vi "produceTimingTicks.vi"(8 "error in (no error)":errorcluster, 10 "Channel":refnum<class "Channel.lvclass">, 11 "RampEvent in":refnum<class "RampEvent.lvclass">) -> (0 "error out":errorcluster, 2 "timingTickList":refnum<class "ScriptEventList.lvclass">, 3 "RampEvent out":refnum<class "RampEvent.lvclass">)   [LabVIEW 2011, in "Tools.lvlib" / "Scripting.lvlib" / "RampEvent.lvclass"]
uses:
  RampEvent.lvclass
  DatabaseHelpers/Database Objects/Channel/Channel.lvclass
  ScriptEventList/ScriptEventList.lvclass
  ScriptEvent.lvclass
panel:
  out "Array":dbl[](array[numeric]) format="%_10g"
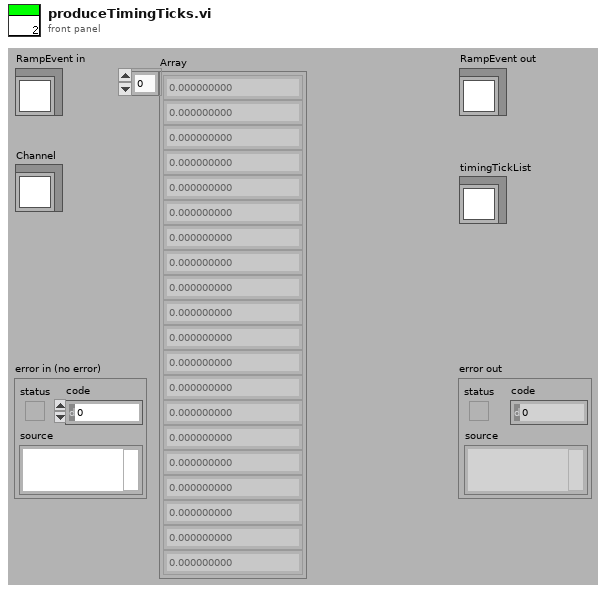
[diagram p1: front panel]
types:
  T1 = enum16{"changeValue", "pulse", "clock", "rampUp", "rampDown", "singleTone", "singleToneRamp", "playFile", "rf", "rfRamp"}
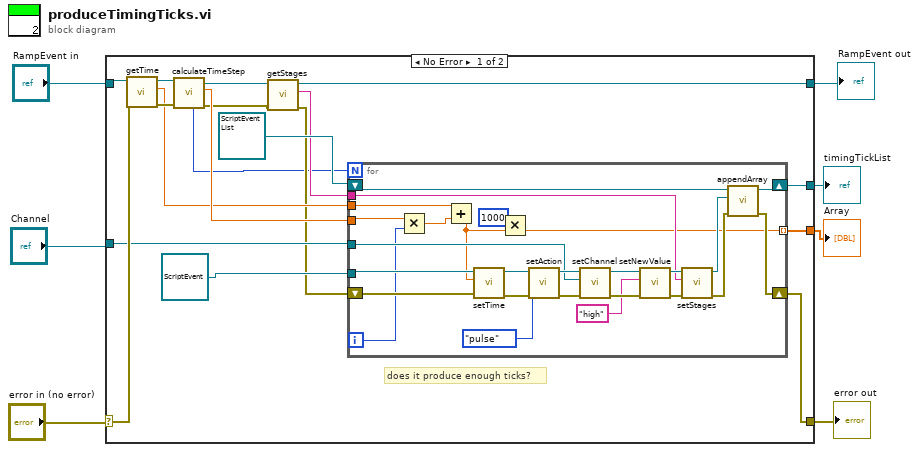
[diagram p0: block diagram]
diagram:
  n1 = case shown="No Error" "error in (no error)" {
    selector: "error in (no error)" -> [w22 w52]
    tunnel: "RampEvent in" -> [w23 w53]
    tunnel: [w18 w52] -> w3
    tunnel: [w10 w53] -> w5
    tunnel: "Channel" -> [w19 _]
    tunnel: [w16 _] -> w2
    tunnel: [w8 _] -> w1
    frame No Error {
      # "does it produce enough ticks?"
      n2 = call "getTime.vi"("error in (no error)"=w22, "ScriptEvent.lvclass in"=w23) -> ("error out"=w21:errorcluster, "time"=w20:dbl, "ScriptEvent.lvclass out"=w24:refnum<class "RampEvent.lvclass">)  [unwired: 7 in]
      n3 = call "calculateTimeStep.vi"("error in (no error)"=w21, "RampEvent in"=w24) -> ("error out"=w13:errorcluster, "timeStep"=w25:dbl, "RampEvent out"=w14:refnum<class "RampEvent.lvclass">, "number of Steps"=w9:i32)  [unwired: 5 in, 1 out]
      n4 = call "getStages.vi"("error in (no error)"=w13, "ScriptEvent.lvclass in"=w14) -> ("error out"=w12:errorcluster, "Stage"=w11:string, "ScriptEvent.lvclass out"=w10:refnum<class "RampEvent.lvclass">)  [unwired: 7 in]
      n5 = for {
        N: w9 -> [_]
        tunnel: w25 -> [w50]
        tunnel: w20 -> [w51]
        tunnel: refnum<class "ScriptEvent.lvclass"> refnum ("Tools.lvlib:Scripting.lvlib:ScriptEvent.lvclass") -> [w48]
        tunnel: w19 -> [w42]
        shift-right: [w35] -> w18
        shift-left: w12 -> [w47]
        shift-right: [w37] -> w16
        shift-left: refnum<class "ScriptEventList.lvclass"> refnum ("Tools.lvlib:Scripting.lvlib:ScriptEventList.lvclass") -> [w36]
        tunnel: w11 -> [w30]
        tunnel: [w27] -> w8 mode=indexing
        i -> [w38]
        n6 = Multiply(x=w50, y=w38) -> (x*y=w49:dbl)
        n7 = Add(x=w51, y=w49) -> (x+y=w28:dbl)
        n8 = call "setTime.vi"("error in (no error)"=w47, "time"=w28, "ScriptEvent.lvclass in"=w48) -> ("error out"=w45:errorcluster, "ScriptEvent.lvclass out"=w46:refnum<class "ScriptEvent.lvclass">)  [unwired: 7 in]
        n9 = Multiply(x=1000, y=w28) -> (x*y=w27:dbl)
        n10 = call "setAction.vi"("error in (no error)"=w45, "action"=T1."pulse", "ScriptEvent.lvclass in"=w46) -> ("error out"=w43:errorcluster, "ScriptEvent.lvclass out"=w44:refnum<class "ScriptEvent.lvclass">)  [unwired: 7 in]
        n11 = call-dynamic "setChannel.vi"("error in (no error)"=w43, "Channel.lvclass"=w42, "ScriptEvent.lvclass in"=w44) -> ("error out"=w40:errorcluster, "ScriptEvent.lvclass out"=w41:refnum<class "ScriptEvent.lvclass">)  [unwired: 7 in]
        n12 = call "setNewValue.vi"("error in (no error)"=w40, "newValue"="high", "ScriptEvent.lvclass in"=w41) -> ("error out"=w33:errorcluster, "ScriptEvent.lvclass out"=w34:refnum<class "ScriptEvent.lvclass">)  [unwired: 7 in]
        n13 = call-dynamic "setStages.vi"("error in (no error)"=w33, "Stage"=w30, "ScriptEvent.lvclass in"=w34) -> ("error out"=w32:errorcluster, "ScriptEvent.lvclass out"=w31:refnum<class "ScriptEvent.lvclass">)  [unwired: 7 in]
        n14 = call "appendArray.vi"("error in (no error)"=w32, "ScriptEvent"=w31, "ScriptEventList in"=w36) -> ("error out"=w35:errorcluster, "ScriptEventList out"=w37:refnum<class "ScriptEventList.lvclass">)  [unwired: 6 in, 1 out]
      }
    }
    frame Error {
    }
  }
  "error out" <- w3
  "RampEvent out" <- w5
  "timingTickList" <- w2
  "Array" <- w1
